vi "Identify Neocera.vi"(7 "Just add \";\"":bool, 8 "error in (no error)":errorcluster, 11 "VISA Resource Name":refnum<visa-resource-name>) -> (0 "error out":errorcluster, 1 "data string out":string, 2 "Identified":bool, 3 "VISA Resource Name Out":refnum<visa-resource-name>)   [LabVIEW 2015]
uses:
  GPIB/VISA  Send Receive.vi
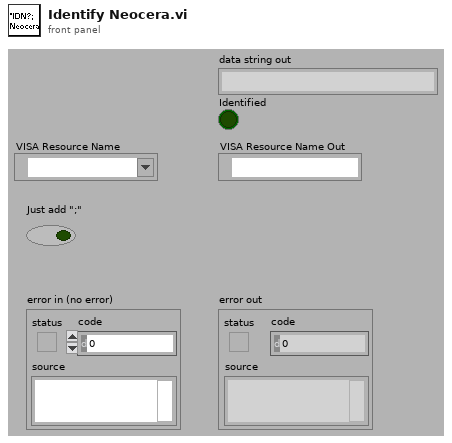
[diagram p1: front panel]
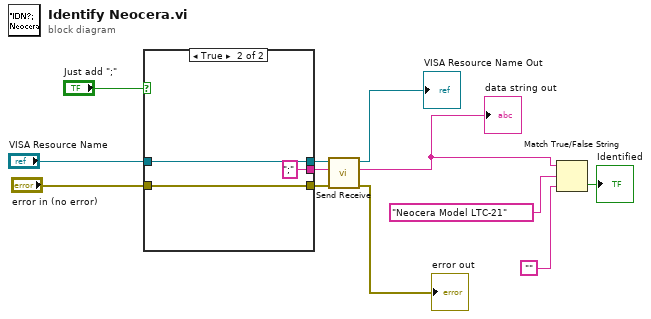
[diagram p0: block diagram]
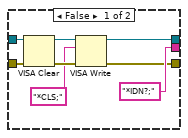
[diagram p2: hidden frame]
diagram:
  n1 = case shown="True" "Just add \";\"" {
    tunnel: "error in (no error)" -> [w20 w23]
    tunnel: ["*IDN?;" ("data string in") ";" ("data string in")] -> w9
    tunnel: "VISA Resource Name" -> [w18 w22]
    tunnel: [w16 w23] -> w3
    tunnel: [w14 w22] -> w2
    frame False {
      n2 = VISA Clear(VISA resource name=w18, error in (no error)=w20) -> (VISA resource name out=w15:refnum<visa-resource-name>, error out=w17:errorcluster)
      n3 = VISA Write(VISA resource name=w15, write buffer="*CLS;", error in (no error)=w17) -> (VISA resource name out=w14:refnum<visa-resource-name>, error out=w16:errorcluster)  [unwired: 1 out]
    }
    frame True {
    }
  }
  n4 = call-poly "Send Receive.vi"("error in (no error)"=w3, "data string in"=w9, "VISA Resource Name"=w2) -> ("error out"=→"error out":errorcluster, "data string out"=w8:string, "VISA Resource Name Out"=→"VISA Resource Name Out":refnum<visa-resource-name>)  [unwired: 6 in]
  "data string out" <- w8
  n5 = Match True/False String(2:"", 3:"Neocera Model LTC-21", 4:w8) -> (0:→"Identified":bool)  [unwired: 1 out]
